vi "PDP MagLocal Message.vi"   [LabVIEW 2009]
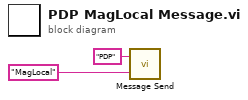
[diagram p0: block diagram]
diagram:
  n1 = call "Message Send.vi"("Message"="MagLocal", "Destination"="PDP") -> ()
